vi "Convert Function Set to Cmd.vi"(7 "8bit":bool=TRUE, 11 "font configuration":T1(ring)) -> (3 "function set cmd code":u8)   [LabVIEW 2015, in "HD44780 FPGA.lvlib"]
uses:
  <vilib>/EmbeddedDisplay/Hitachi HD44780/FPGA/HD44780 FPGA.lvlib
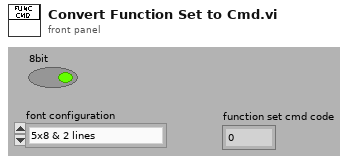
[diagram p1: front panel]
types:
  T1 = enum8{"5x8 & 2 lines", "5x10 & 1 line", "5x8 & 1 line"}
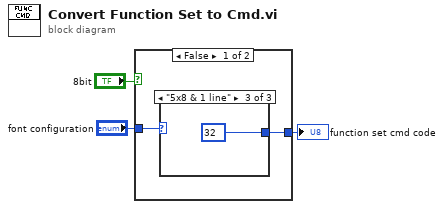
[diagram p0: block diagram]
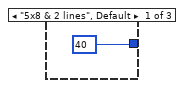
[diagram p2: hidden frame]
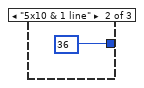
[diagram p3: hidden frame]
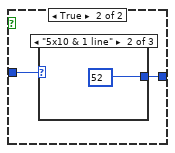
[diagram p4: hidden frame]
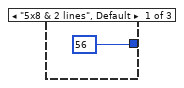
[diagram p5: hidden frame]
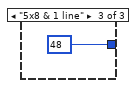
[diagram p6: hidden frame]
diagram:
  n1 = case shown="False" "8bit" {
    tunnel: [w4 w10] -> w3
    tunnel: "font configuration" -> [w5 w9]
    frame False {
      n2 = case shown="\"5x8 & 1 line\"" w5 {
        tunnel: [u8 40 ("LCD data/cmd") u8 36 ("LCD data/cmd") u8 32 ("LCD data/cmd")] -> w4
        frame "5x8 & 2 lines", Default {
        }
        frame "5x10 & 1 line" {
        }
        frame "5x8 & 1 line" {
        }
      }
    }
    frame True {
      n3 = case shown="\"5x10 & 1 line\"" w9 {
        tunnel: [u8 56 ("LCD data/cmd") u8 52 ("LCD data/cmd") u8 48 ("LCD data/cmd")] -> w10
        frame "5x8 & 2 lines", Default {
        }
        frame "5x10 & 1 line" {
        }
        frame "5x8 & 1 line" {
        }
      }
    }
  }
  "function set cmd code" <- w3
